vi "assembly_tray_region.vi"() -> ()   [LabVIEW 2021]
panel:
  out "Assembly Tray Region":dbl
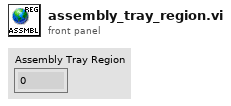
[diagram p1: front panel]
diagram:
